vi "main.vi"() -> ()   [LabVIEW 2012]
uses:
  PCI9757_32.dll
panel:
  out "导入文件大小":dbl
  out "通道使能数组":dbl[](array[numeric])
  out "通道量程数组":dbl[](array[numeric])
  out "通道总数":dbl
  out "数组":path[](array[path])
  in  "退出系统":bool
  in  "选项卡控件":enum32{"AD采集", "数据回放"}(tab)
  in  "时钟源选择":u16(ring) items=["内部时钟", "外部时钟"]
  in  "触发方向":u16(ring) items=["负向触发", "正向触发", "正负向触发"]
  in  "触发类型":u16(ring) items=["边沿触发", "脉冲触发"]
  in  "触发源信号":u16(ring) items=["ATR触发", "DTR触发源"]
  in  "触发模式":u16(ring) items=["软件内触发", "硬件后触发"]
  out "混合信号图":dbl[][](graph)
  in  "通道3":bool
  in  "通道2":bool
  in  "通道1":bool
  in  "通道0":bool
  in  "停止AD":bool
  in  "开始AD":bool
  in  "存储":bool
  out "状态":u8(slide) scale=0.0..10.0
  in  "通道0量程":u16(ring) items=["-10000mV~+10000mV", "-5000mV~+5000mV", "-2500mV~+2500mV", "0-10000mV", "0-5000mV"]
  in  "通道3量程":u16(ring) items=["-10000mV~10000mV", "-5000mV~+5000mV", "-2500mV~+2500mV", "0-10000mV", "0-5000mV"]
  in  "通道1量程":u16(ring) items=["-10000mV~+10000mV", "-5000mV~+5000mV", "-2500mV~+2500mV", "0-10000mV", "0-5000mV"]
  in  "通道2量程":u16(ring) items=["-10000mV~+10000mV", "-5000mV~+5000mV", "-2500mV~+2500mV", "0-10000mV", "0-5000mV"]
  in  "文件名":string
  in  "触发电平":u32
  in  "触发灵敏窗":u32=40
  in  "测试功能":enum16{"非空", "半满", "DMA"}(ring)
  in  "采样频率":u32=10000
  in  "导入":bool
  out "Waveform Graph 3":dynamicdata(graph)
  in  "开始":bool
  in  "刷新速度":u32(knob)=100 min=100 max=1000 step=100 scale=100.0..1000.0
  in  "显示点数":u32(knob)=1000 min=1 max=10000 step=1000 scale=1.0..10000.0
  in  "量程输入":i32(ring) items=["±10000mV", "±5000mV", "±2500mV", "0-10000mV", "0-5000mV"]
  # "通道使能"
  # "通道量程"
  # "mV"
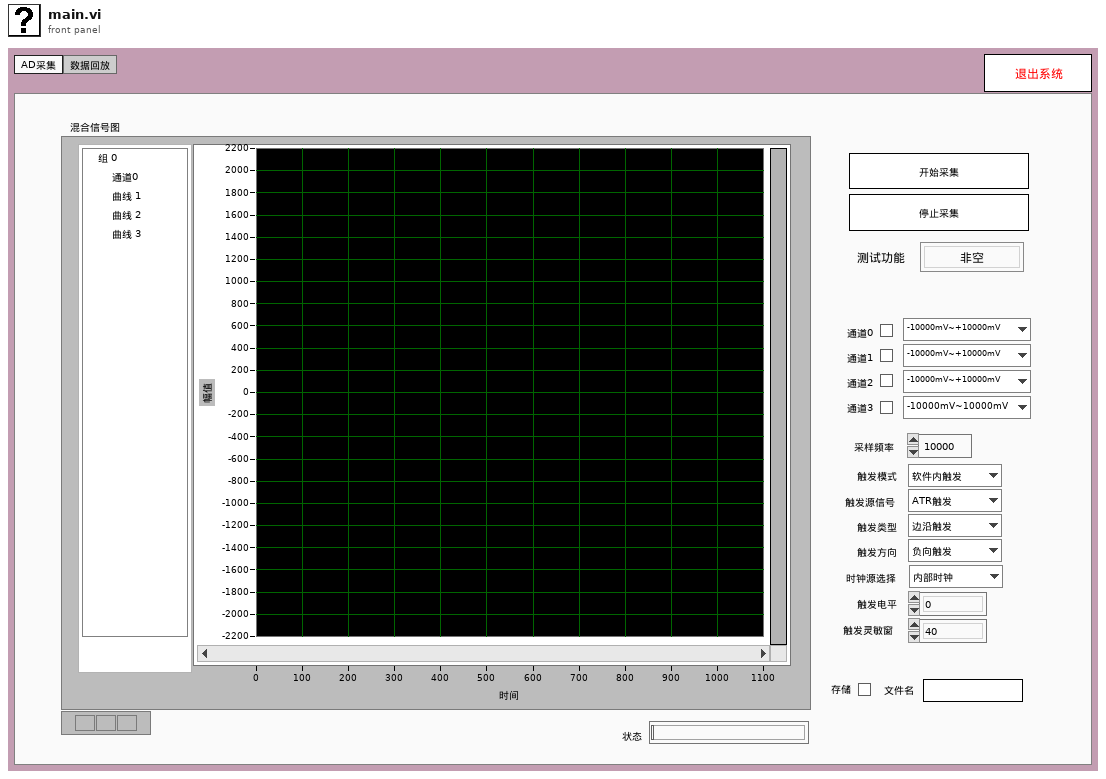
[diagram p1: front panel]
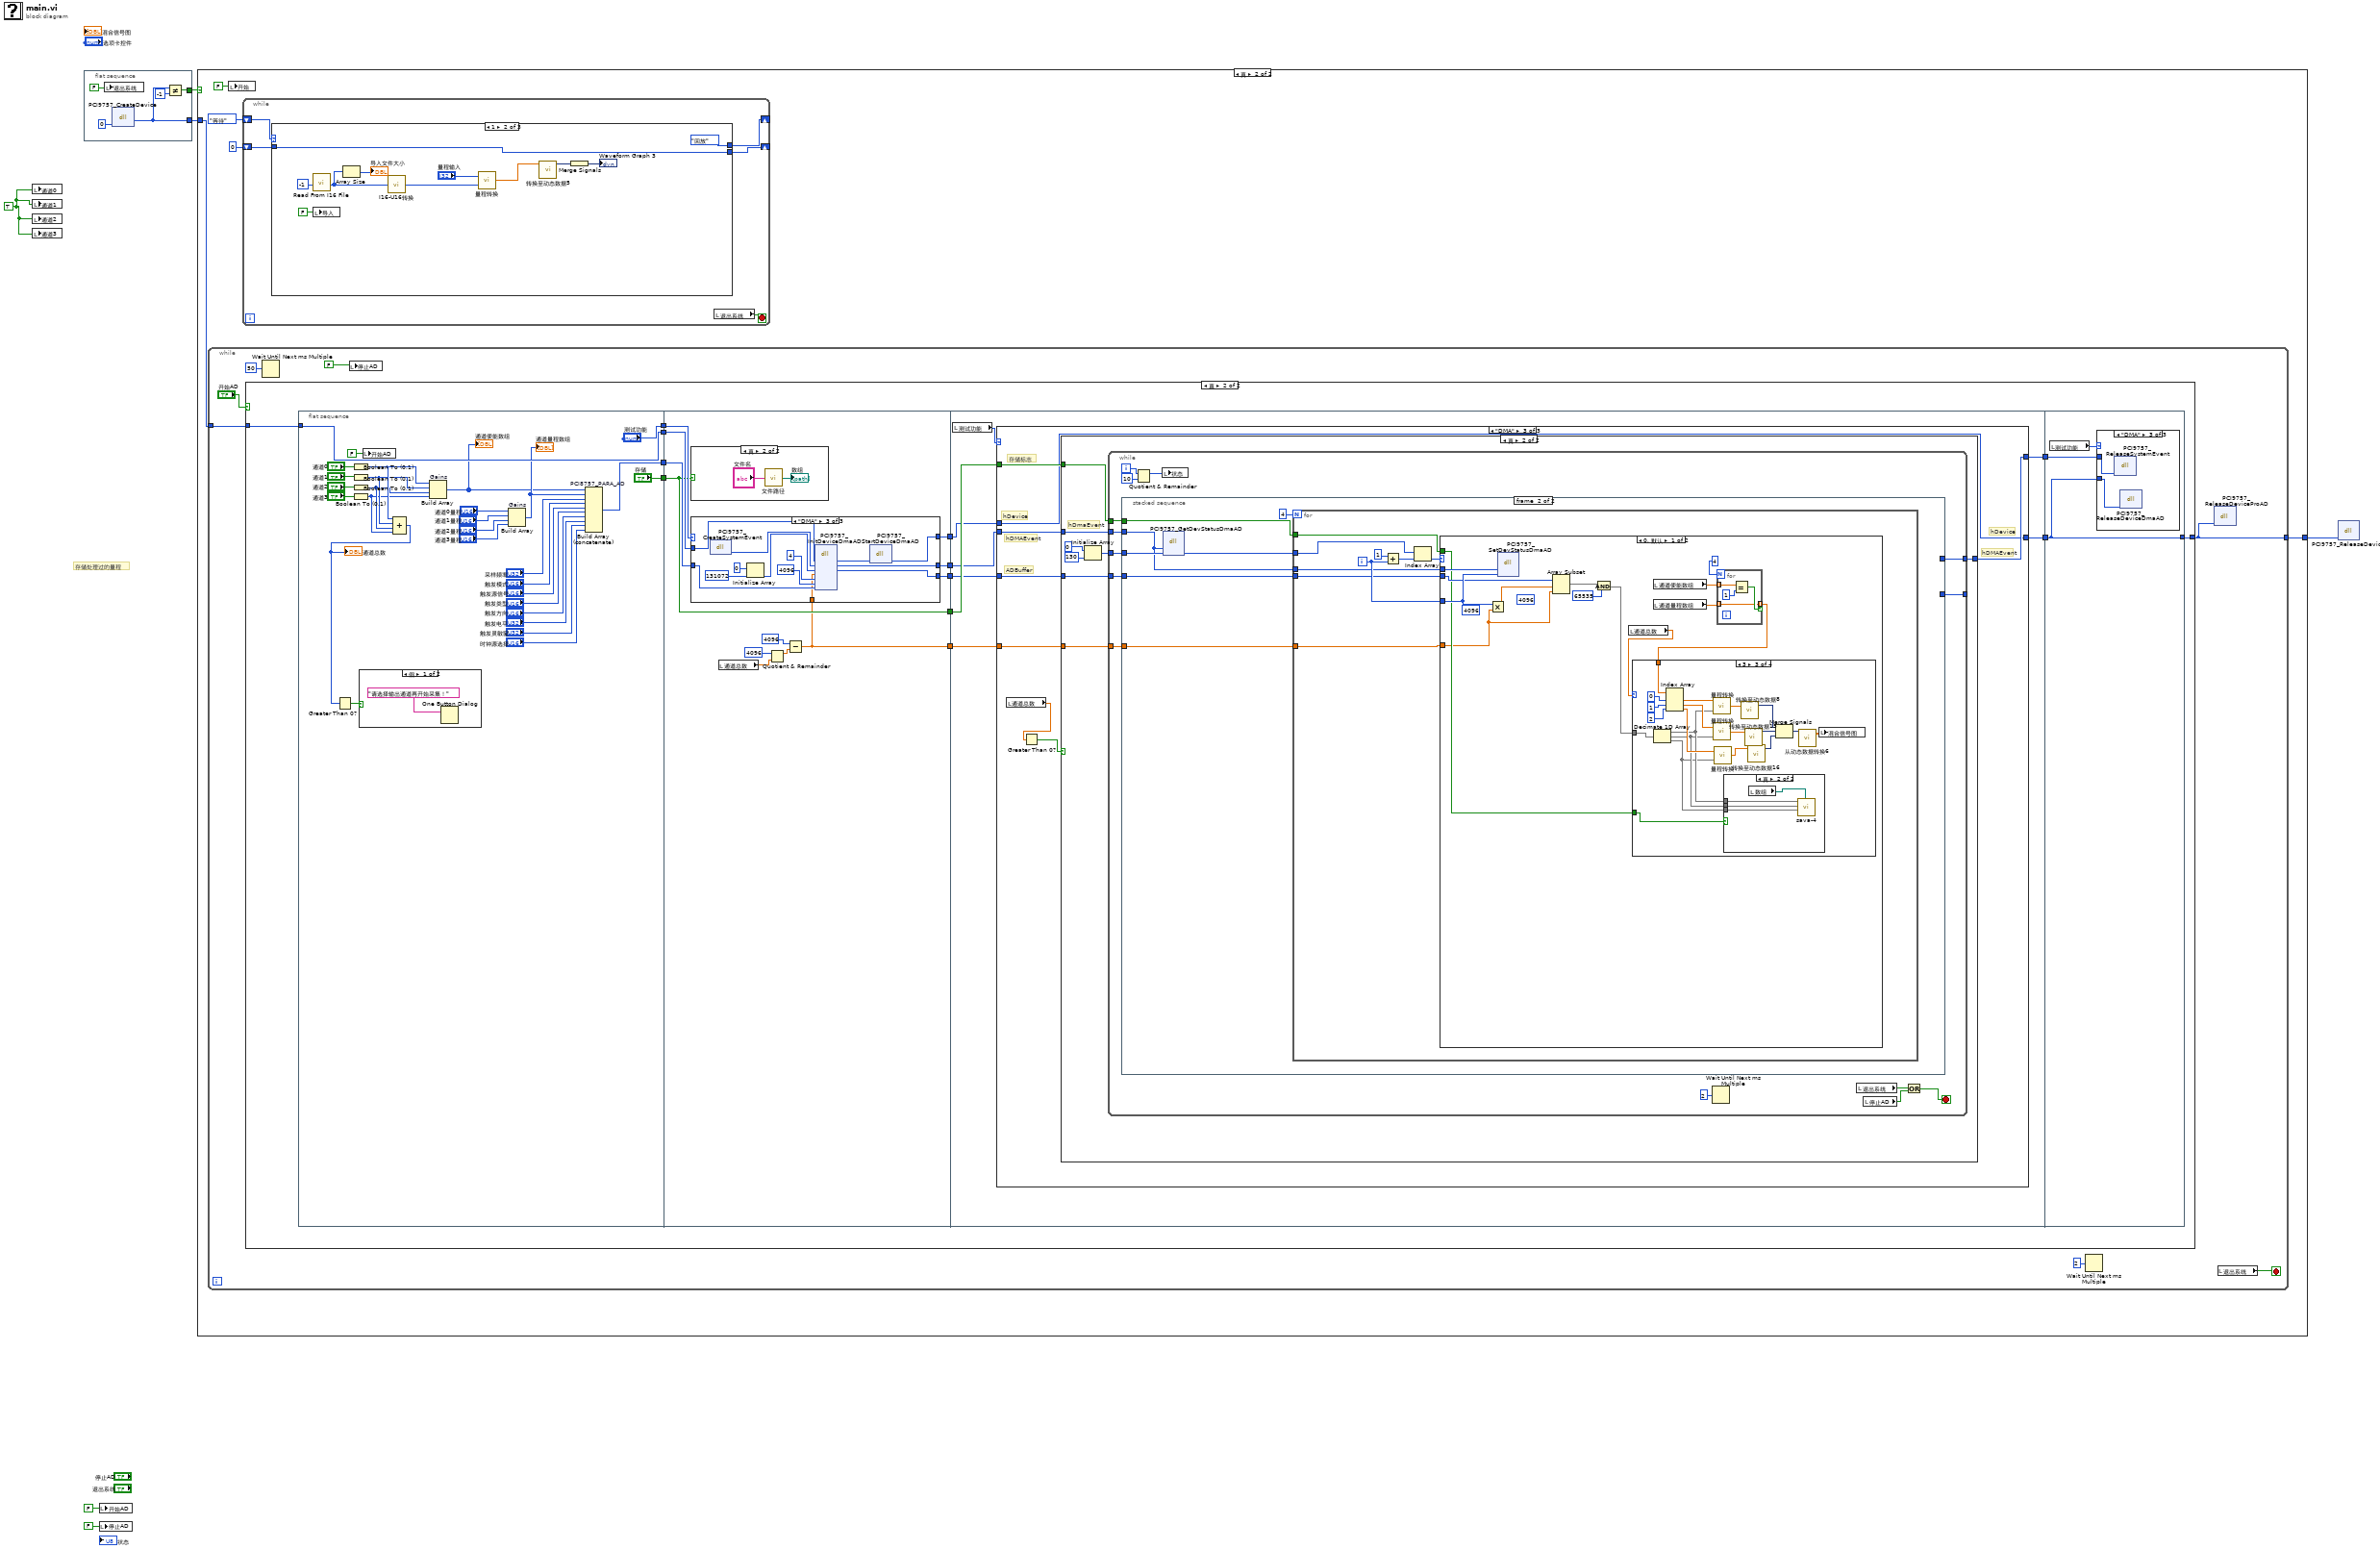
[diagram p0: block diagram]
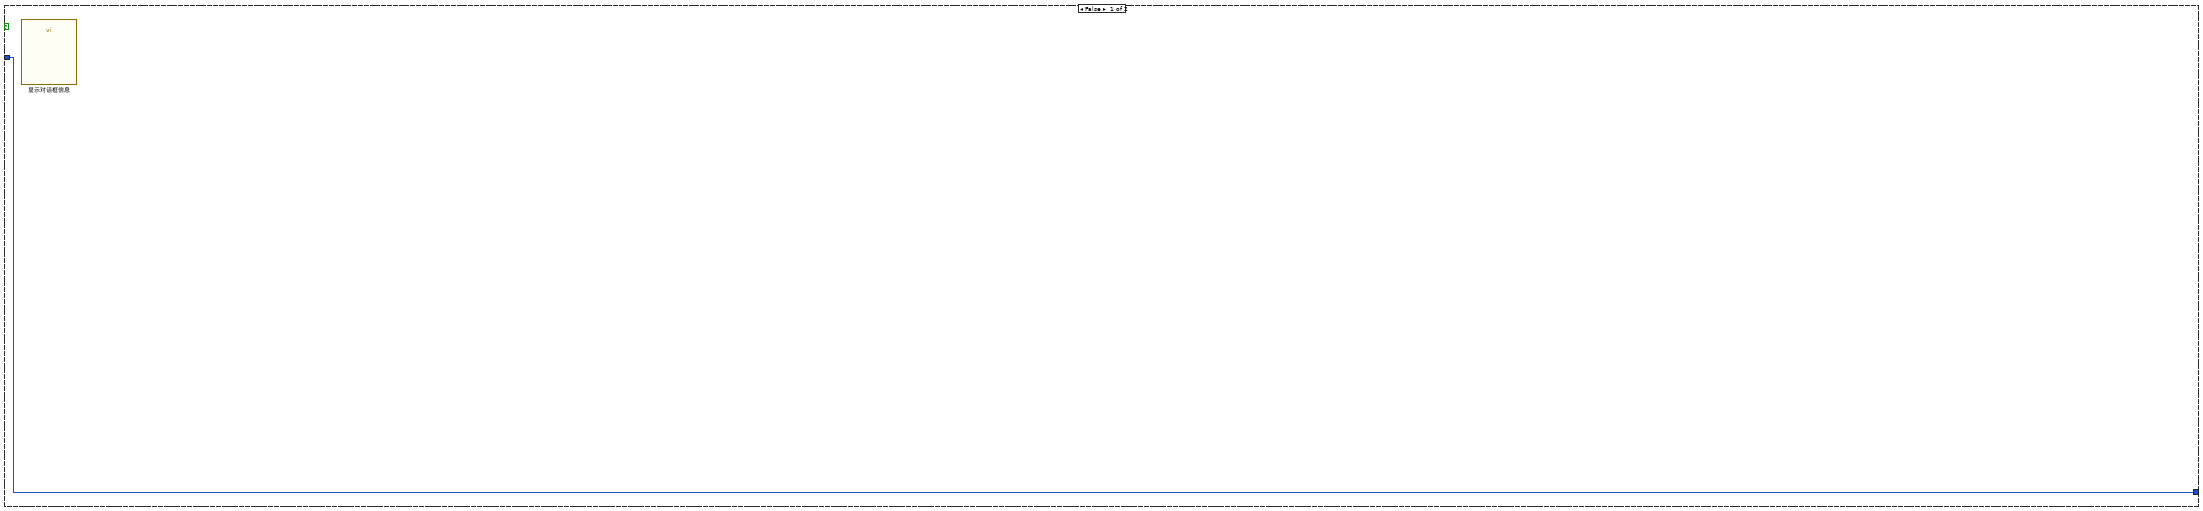
[diagram p2: hidden frame]
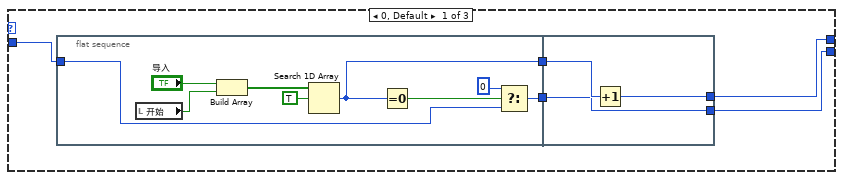
[diagram p3: hidden frame]
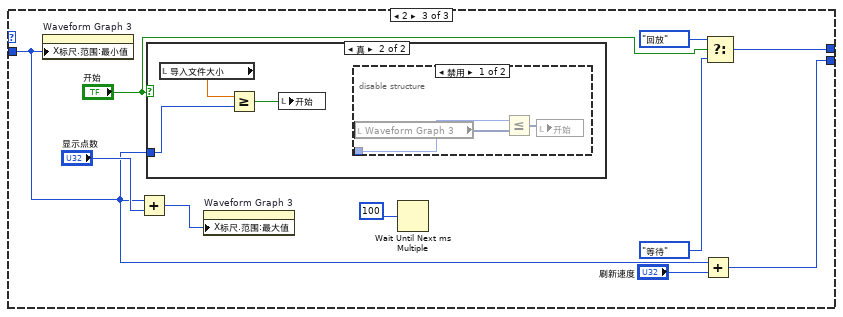
[diagram p4: hidden frame]
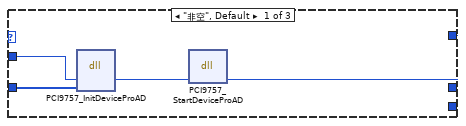
[diagram p10: hidden frame]
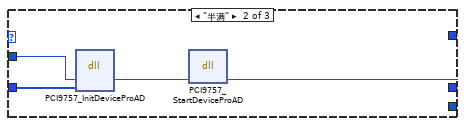
[diagram p11: hidden frame]
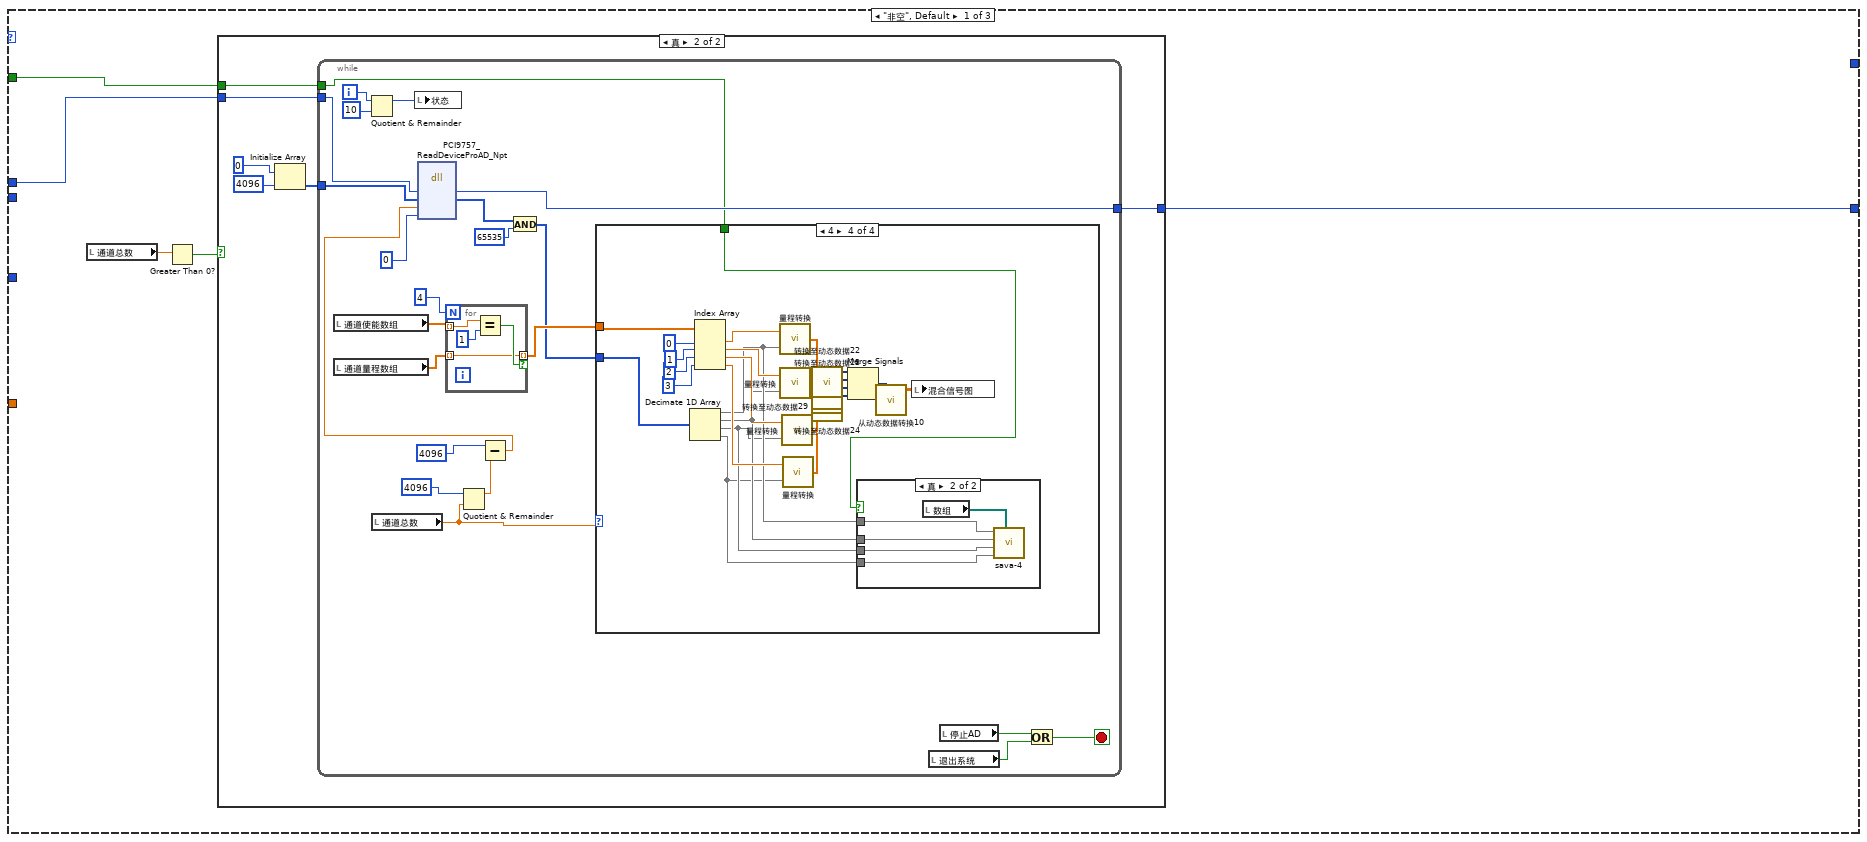
[diagram p12: hidden frame]
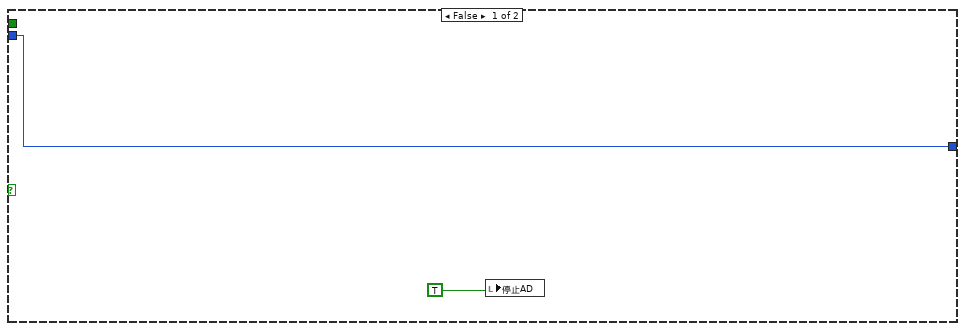
[diagram p13: hidden frame]
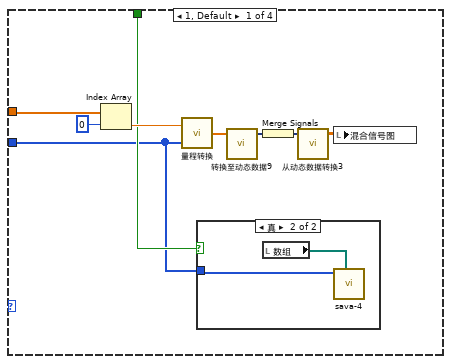
[diagram p14: hidden frame]
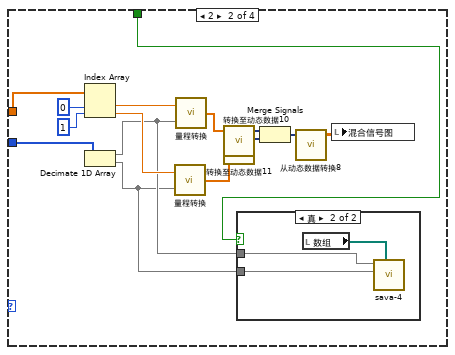
[diagram p16: hidden frame]
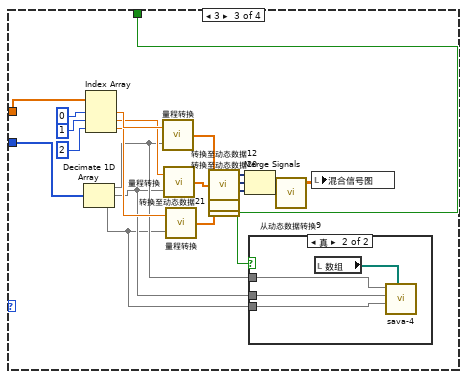
[diagram p18: hidden frame]
diagram:
  w1 = TRUE
  # "存储处理过的量程"
  n1 = local write "通道0"(w1) -> ()
  n2 = local write "通道1"(w1) -> ()
  n3 = local write "通道2"(w1) -> ()
  n4 = local write "通道3"(w1) -> ()
  n5 = flat-sequence {
    tunnel: [w10] -> w4
    tunnel: [w8] -> w3
    frame #0 {
      n6 = local write "退出系统"(FALSE ("退出系统")) -> ()
      n7 = dll-call lib="PCI9757_32.dll" fn="PCI9757_CreateDevice" label="CreateDevice"("DeviceID"=0) -> ("返回类型"=w8:i32)  [unwired: 4 in, 2 out]
      n8 = Not Equal?(x=w8, y=-1) -> (x != y?=w10:bool)
    }
  }
  n9 = local write "开始AD"(FALSE ("开始AD")) -> ()
  n10 = local write "停止AD"(FALSE ("停止AD")) -> ()
  n11 = case shown="真" w4 {
    tunnel: w3 -> [w12 w14]
    tunnel: [w12 w13] -> w2
    frame False {
      n12 = call "显示对话框信息"() -> ()  [unwired: 10 in, 2 out]
    }
    frame True {
      n13 = while {
        tunnel: w14 -> [w70]
        tunnel: [w69] -> w13
        stop <- w71 stop-if-true
        n14 = case shown="真" "开始AD" {
          tunnel: w70 -> [w74 w82]
          tunnel: [w74 w80] -> w69
          frame False {
          }
          frame True {
            n15 = flat-sequence {
              tunnel: ["测试功能"] -> w87
              tunnel: ["存储"] -> w85
              tunnel: [w109] -> w84
              tunnel: [w114] -> w83
              tunnel: w82 -> [w114]
              tunnel: [w124] -> w86
              tunnel: w87 -> [w129]
              tunnel: w85 -> [w123]
              tunnel: w84 -> [w128]
              tunnel: w83 -> [w127]
              tunnel: [w123] -> w79
              tunnel: [w126] -> w78
              tunnel: [w125] -> w77
              tunnel: [w118] -> w75
              tunnel: w86 -> [w158]
              tunnel: [w160] -> w81
              tunnel: w79 -> [w159]
              tunnel: w78 -> [w157]
              tunnel: w77 -> [w156]
              tunnel: [w154] -> w76
              tunnel: w75 -> [w153]
              tunnel: w81 -> [w588]
              tunnel: [w588] -> w80
              tunnel: w76 -> [w587]
              frame #0 {
                n16 = Boolean To (0,1)(Boolean="通道0") -> (0, 1=w96:i16)
                n17 = Boolean To (0,1)(Boolean="通道1") -> (0, 1=w95:i16)
                n18 = Boolean To (0,1)(Boolean="通道2") -> (0, 1=w94:i16)
                n19 = Boolean To (0,1)(Boolean="通道3") -> (0, 1=w93:i16)
                n20 = local write "开始AD"(FALSE ("开始AD")) -> ()
                n21 = Compound Arithmetic op=ADD(w96, w95, w94, w93) -> (w92:i16)
                "通道总数" <- w92
                n22 = Greater Than 0?(x=w92) -> (x > 0?=w97:bool)
                n23 = case shown="假" w97 {
                  frame False {
                    n24 = One Button Dialog(message="请选择输出通道再开始采集！") -> ()  [unwired: 1 in, 1 out]
                  }
                  frame True {
                  }
                }
                n25 = Build Array "Gains"(w96, w95, w94, w93) -> (w90:i16[])
                "通道使能数组" <- w90
                n26 = Build Array "Gains"("通道0量程", "通道1量程", "通道2量程", "通道3量程") -> (w91:u16[])
                "通道量程数组" <- w91
                n27 = Build Array (concatenate) "PCI8757_PARA_AD"(w90, w91, "采样频率", "触发模式", "触发源信号", "触发类型", "触发方向", "触发电平", "触发灵敏窗", "时钟源选择") -> (w109:u32[])
              }
              frame #1 {
                n28 = case shown="真" w123 {
                  frame False {
                  }
                  frame True {
                    n29 = call "文件路径.vi"("文件名"="文件名") -> ("数组"=→"数组":path[])
                  }
                }
                n30 = local read "通道总数"() -> (w120:dbl)
                n31 = Quotient & Remainder(x=4096 ("nReadSizeWords"), y=w120) -> (x-y*floor(x/y)=w119:dbl)  [unwired: 1 out]
                n32 = Subtract(x=4096 ("nReadSizeWords"), y=w119) -> (x-y=w118:dbl)
                n33 = case shown="\"DMA\"" w129 {
                  tunnel: w128 -> [w133 w137 w143]
                  tunnel: w127 -> [w134 w138 w141]
                  tunnel: [_ _ w145] -> w126
                  tunnel: [_ _ w144] -> w125
                  tunnel: [w132 w136 w142] -> w124
                  tunnel: w118 -> [_ _ w140]
                  frame "非空", Default {
                    n34 = dll-call lib="PCI9757_32.dll" fn="PCI9757_InitDeviceProAD" label="InitDeviceProAD"("hDevice"=w134, "pAPara"=w133) -> ("hDevice"=w135:i32)  [unwired: 5 in, 2 out]
                    n35 = dll-call lib="PCI9757_32.dll" fn="PCI9757_StartDeviceProAD" label="StartDeviceProAD"("hDevice"=w135) -> ("hDevice"=w132:i32)  [unwired: 4 in, 2 out]
                  }
                  frame "半满" {
                    n36 = dll-call lib="PCI9757_32.dll" fn="PCI9757_InitDeviceProAD" label="InitDeviceProAD"("hDevice"=w138, "pAPara"=w137) -> ("hDevice"=w139:i32)  [unwired: 5 in, 2 out]
                    n37 = dll-call lib="PCI9757_32.dll" fn="PCI9757_StartDeviceProAD" label="StartDeviceProAD"("hDevice"=w139) -> ("hDevice"=w136:i32)  [unwired: 4 in, 2 out]
                  }
                  frame "DMA" {
                    n38 = dll-call lib="PCI9757_32.dll" fn="PCI9757_CreateSystemEvent" label="CreateSystemEvent"() -> ("hEvent"=w149:i32)  [unwired: 3 in, 2 out]
                    n39 = Initialize Array(0, 131072 ("dimension size")) -> (w148:i32[])
                    n40 = dll-call lib="PCI9757_32.dll" fn="PCI9757_InitDeviceDmaAD" label="InitDeviceDmaAD"("hDevice"=w141, "hDmaEvent"=w149, "ADBuffer"=w148, "nReadSizeWords"=w140, "nSegmentCount"=4, "nSegmentSizeWords"=4096, "pADPara"=w143) -> ("hDevice"=w152:i32, "hDmaEvent"=w145:i32, "ADBuffer"=w144:u32[])  [unwired: 8 in, 2 out]
                    n41 = dll-call lib="PCI9757_32.dll" fn="PCI9757_StartDeviceDmaAD" label="StartDeviceDmaAD"("hDevice"=w152) -> ("hDevice"=w142:i32)  [unwired: 4 in, 2 out]
                  }
                }
              }
              frame #2 {
                n42 = local read "测试功能"() -> (w155:enum16{"非空", "半满", "DMA"})
                n43 = case shown="\"DMA\"" w155 {
                  tunnel: w158 -> [w165 w287 w430]
                  tunnel: [w164 w284 w430] -> w160
                  tunnel: w159 -> [w163 w288 w431]
                  tunnel: w157 -> [_ _ w433]
                  tunnel: w156 -> [_ _ w429]
                  tunnel: [_ _ w432] -> w154
                  tunnel: w153 -> [_ _ w426]
                  frame "非空", Default {
                    n44 = local read "通道总数"() -> (w162:dbl)
                    n45 = Greater Than 0?(x=w162) -> (x > 0?=w161:bool)
                    n46 = case shown="真" w161 {
                      tunnel: w165 -> [w167 w170]
                      tunnel: [w167 w169] -> w164
                      tunnel: w163 -> [_ w168]
                      frame False {
                        n47 = local write "停止AD"(TRUE) -> ()
                      }
                      frame True {
                        n48 = Initialize Array(0, 4096 ("dimension size")) -> (w171:i32[])
                        n49 = while {
                          tunnel: w171 -> [w188]
                          tunnel: w170 -> [w187]
                          tunnel: [w186] -> w169
                          tunnel: w168 -> [w179]
                          i -> [w192]
                          stop <- w194 stop-if-true
                          n50 = local read "通道使能数组"() -> (w183:dbl[])
                          n51 = local read "通道量程数组"() -> (w182:dbl[])
                          n52 = Quotient & Remainder(x=w192, y=10) -> (x-y*floor(x/y)=w191:i32)  [unwired: 1 out]
                          n53 = local read "通道总数"() -> (w177:dbl)
                          n54 = local write "状态"(w191) -> ()
                          n55 = for {
                            N: 4 -> [_]
                            tunnel: w183 -> [w283] mode=indexing
                            tunnel: w182 -> [w280] mode=indexing
                            tunnel: [w280] -> w181 mode=indexing if=w281
                            n56 = Equal?(x=w283, y=1) -> (x = y?=w281:bool)
                          }
                          n57 = Quotient & Remainder(x=4096, y=w177) -> (x-y*floor(x/y)=w176:dbl)  [unwired: 1 out]
                          n58 = Subtract(x=4096, y=w176) -> (x-y=w174:dbl)
                          n59 = dll-call lib="PCI9757_32.dll" fn="PCI9757_ReadDeviceProAD_Npt" label="ReadDeviceProAD_Npt"("hDevice"=w187, "ADBuffer"=w188, "nReadSizeWords"=w174, "nRetSizeWords"=0) -> ("hDevice"=w186:i32, "ADBuffer"=w185:u32[])  [unwired: 6 in, 2 out]
                          n60 = And(x=w185, y=65535) -> (x .and. y?=w180:u32[])
                          n61 = case shown="4" w177 {
                            tunnel: w181 -> [w205 w222 w245 w274]
                            tunnel: w180 -> [w197 w219 w241 w269]
                            tunnel: w179 -> [w198 w208 w226 w250]
                            frame 1, Default {
                              n62 = Index Array(array=w205, index=0) -> (element=w203:dbl)
                              n63 = call "量程转换.vi"("输入"=w197, "量程输入"=w203) -> ("输出"=w200:dbl[])
                              n64 = case shown="真" w198 {
                                tunnel: w197 -> [_ w206]
                                frame False {
                                }
                                frame True {
                                n65 = local read "数组"() -> (w207:path[])
                                n66 = call "sava-4.vi"("datafile"=w207, "1D array"=w206) -> ()  [unwired: 10 in]
                                }
                              }
                              n67 = call "转换至动态数据9"("Array"=w200) -> ("Dynamic Data Type"=w199:dynamicdata)  [unwired: 3 in]
                              n68 = Merge Signals(w199) -> (w202:dynamicdata)
                              n69 = call "从动态数据转换3"("Dynamic Data Type"=w202) -> ("Array"=w201:dbl[][])  [unwired: 3 in]
                              n70 = local write "混合信号图"(w201) -> ()
                            }
                            frame 2 {
                              n71 = Index Array(array=w222, index #1=0, index #2=1) -> (element #1=w218:dbl, element #2=w217:dbl)
                              n72 = Decimate 1D Array(w219) -> (w210:u32[], w209:u32[])
                              n73 = call "量程转换.vi"("输入"=w209, "量程输入"=w217) -> ("输出"=w214:dbl[])
                              n74 = call "量程转换.vi"("输入"=w210, "量程输入"=w218) -> ("输出"=w216:dbl[])
                              n75 = call "转换至动态数据10"("Array"=w216) -> ("Dynamic Data Type"=w215:dynamicdata)  [unwired: 3 in]
                              n76 = call "转换至动态数据11"("Array"=w214) -> ("Dynamic Data Type"=w213:dynamicdata)  [unwired: 3 in]
                              n77 = case shown="真" w208 {
                                tunnel: w210 -> [_ w224]
                                tunnel: w209 -> [_ w223]
                                frame False {
                                }
                                frame True {
                                n78 = local read "数组"() -> (w225:path[])
                                n79 = call "sava-4.vi"("datafile"=w225, "1D array 2"=w223, "1D array"=w224) -> ()  [unwired: 9 in]
                                }
                              }
                              n80 = Merge Signals(w215, w213) -> (w212:dynamicdata)
                              n81 = call "从动态数据转换8"("Dynamic Data Type"=w212) -> ("Array"=w211:dbl[][])  [unwired: 3 in]
                              n82 = local write "混合信号图"(w211) -> ()
                            }
                            frame 3 {
                              n83 = Decimate 1D Array(w241) -> (w229:u32[], w228:u32[], w227:u32[])
                              n84 = Index Array(array=w245, index #1=0, index #2=1, index #3=2) -> (element #1=w240:dbl, element #2=w239:dbl, element #3=w238:dbl)
                              n85 = call "量程转换.vi"("输入"=w229, "量程输入"=w240) -> ("输出"=w237:dbl[])
                              n86 = call "量程转换.vi"("输入"=w228, "量程输入"=w239) -> ("输出"=w235:dbl[])
                              n87 = call "量程转换.vi"("输入"=w227, "量程输入"=w238) -> ("输出"=w233:dbl[])
                              n88 = call "转换至动态数据12"("Array"=w237) -> ("Dynamic Data Type"=w236:dynamicdata)  [unwired: 3 in]
                              n89 = call "转换至动态数据20"("Array"=w235) -> ("Dynamic Data Type"=w234:dynamicdata)  [unwired: 3 in]
                              n90 = call "转换至动态数据21"("Array"=w233) -> ("Dynamic Data Type"=w232:dynamicdata)  [unwired: 3 in]
                              n91 = Merge Signals(w236, w234, w232) -> (w231:dynamicdata)
                              n92 = case shown="真" w226 {
                                tunnel: w229 -> [_ w248]
                                tunnel: w228 -> [_ w247]
                                tunnel: w227 -> [_ w246]
                                frame False {
                                }
                                frame True {
                                n93 = local read "数组"() -> (w249:path[])
                                n94 = call "sava-4.vi"("datafile"=w249, "1D array 3"=w246, "1D array 2"=w247, "1D array"=w248) -> ()  [unwired: 8 in]
                                }
                              }
                              n95 = call "从动态数据转换9"("Dynamic Data Type"=w231) -> ("Array"=w230:dbl[][])  [unwired: 3 in]
                              n96 = local write "混合信号图"(w230) -> ()
                            }
                            frame 4 {
                              n97 = Decimate 1D Array(w269) -> (w254:u32[], w253:u32[], w252:u32[], w251:u32[])
                              n98 = Index Array(array=w274, index #1=0, index #2=1, index #3=2, index #4=3) -> (element #1=w268:dbl, element #2=w267:dbl, element #3=w266:dbl, element #4=w265:dbl)
                              n99 = call "量程转换.vi"("输入"=w254, "量程输入"=w268) -> ("输出"=w264:dbl[])
                              n100 = call "量程转换.vi"("输入"=w253, "量程输入"=w267) -> ("输出"=w262:dbl[])
                              n101 = call "量程转换.vi"("输入"=w252, "量程输入"=w266) -> ("输出"=w260:dbl[])
                              n102 = call "量程转换.vi"("输入"=w251, "量程输入"=w265) -> ("输出"=w258:dbl[])
                              n103 = call "转换至动态数据22"("Array"=w264) -> ("Dynamic Data Type"=w263:dynamicdata)  [unwired: 3 in]
                              n104 = call "转换至动态数据23"("Array"=w262) -> ("Dynamic Data Type"=w261:dynamicdata)  [unwired: 3 in]
                              n105 = call "转换至动态数据24"("Array"=w260) -> ("Dynamic Data Type"=w259:dynamicdata)  [unwired: 3 in]
                              n106 = call "转换至动态数据29"("Array"=w258) -> ("Dynamic Data Type"=w257:dynamicdata)  [unwired: 3 in]
                              n107 = Merge Signals(w263, w261, w259, w257) -> (w256:dynamicdata)
                              n108 = case shown="真" w250 {
                                tunnel: w254 -> [_ w278]
                                tunnel: w253 -> [_ w277]
                                tunnel: w252 -> [_ w276]
                                tunnel: w251 -> [_ w275]
                                frame False {
                                }
                                frame True {
                                n109 = local read "数组"() -> (w279:path[])
                                n110 = call "sava-4.vi"("datafile"=w279, "1D array 4"=w275, "1D array 3"=w276, "1D array 2"=w277, "1D array"=w278) -> ()  [unwired: 7 in]
                                }
                              }
                              n111 = call "从动态数据转换10"("Dynamic Data Type"=w256) -> ("Array"=w255:dbl[][])  [unwired: 3 in]
                              n112 = local write "混合信号图"(w255) -> ()
                            }
                          }
                          n113 = local read "退出系统"() -> (w196:bool)
                          n114 = local read "停止AD"() -> (w195:bool)
                          n115 = Or(x=w195, y=w196) -> (x .or. y?=w194:bool)
                        }
                      }
                    }
                  }
                  frame "半满" {
                    n116 = local read "通道总数"() -> (w285:dbl)
                    n117 = Greater Than 0?(x=w285) -> (x > 0?=w286:bool)
                    n118 = case shown="真" w286 {
                      tunnel: w288 -> [_ w293]
                      tunnel: w287 -> [w290 w292]
                      tunnel: [w290 w291] -> w284
                      frame False {
                        n119 = local write "停止AD"(TRUE) -> ()
                      }
                      frame True {
                        n120 = Initialize Array(0, 4096 ("dimension size")) -> (w294:i32[])
                        n121 = while {
                          tunnel: w292 -> [w301]
                          tunnel: w294 -> [w300]
                          tunnel: w293 -> [w299]
                          tunnel: [w297] -> w291
                          i -> [w303]
                          stop <- w306 stop-if-true
                          n122 = stacked-sequence {
                            tunnel: [_ w336] -> w297
                            tunnel: w301 -> [w307 w335]
                            tunnel: w300 -> [_ w334]
                            tunnel: w299 -> [_ w323]
                            frame #0 {
                              n123 = Initialize Array(0, 3) -> (w308:i32[])
                              n124 = while {
                                tunnel: w308 -> [w317]
                                tunnel: w307 -> [w311]
                                stop <- w312 stop-if-true
                                n125 = dll-call lib="PCI9757_32.dll" fn="PCI9757_GetDevStatusProAD" label="GetDevStatusProAD"("hDevice"=w311, "ADStatus"=w317) -> ("ADStatus"=w315:i32[])  [unwired: 5 in, 2 out]
                                n126 = Index Array(array=w315, index=2) -> (element=w314:i32)
                                n127 = Equal?(x=w314, y=1) -> (x = y?=w312:bool)
                              }
                            }
                            frame #1 {
                              n128 = local read "通道总数"() -> (w319:dbl)
                              n129 = Quotient & Remainder(x=4096, y=w319) -> (x-y*floor(x/y)=w321:dbl)  [unwired: 1 out]
                              n130 = Subtract(x=4096, y=w321) -> (x-y=w318:dbl)
                              n131 = Wait Until Next ms Multiple(millisecond multiple=u32 10) -> ()  [unwired: 1 out]
                              n132 = dll-call lib="PCI9757_32.dll" fn="PCI9757_ReadDeviceProAD_Half" label="ReadDeviceProAD_Half"("hDevice"=w335, "ADBuffer"=w334, "nReadSizeWords"=w318, "nRetSizeWords"=0) -> ("hDevice"=w336:i32, "ADBuffer"=w331:u32[])  [unwired: 6 in, 2 out]
                              n133 = local read "通道使能数组"() -> (w328:dbl[])
                              n134 = local read "通道量程数组"() -> (w327:dbl[])
                              n135 = Array Subset(array=w331, index=0, length=w318) -> (w330:u32[])
                              n136 = for {
                                N: 4 -> [_]
                                tunnel: w328 -> [w425] mode=indexing
                                tunnel: w327 -> [w422] mode=indexing
                                tunnel: [w422] -> w325 mode=indexing if=w423
                                n137 = Equal?(x=w425, y=1) -> (x = y?=w423:bool)
                              }
                              n138 = And(x=w330, y=65535) -> (x .and. y?=w324:u32[])
                              n139 = local read "通道总数"() -> (w326:dbl)
                              n140 = case shown="4" w326 {
                                tunnel: w325 -> [w347 w364 w387 w416]
                                tunnel: w324 -> [w340 w359 w383 w411]
                                tunnel: w323 -> [w339 w350 w368 w396]
                                frame 1, Default {
                                n141 = Index Array(array=w347, index=0) -> (element=w345:dbl)
                                n142 = call "量程转换.vi"("输入"=w340, "量程输入"=w345) -> ("输出"=w344:dbl[])
                                n143 = case shown="真" w339 {
                                tunnel: w340 -> [_ w348]
                                frame False {
                                }
                                frame True {
                                n144 = local read "数组"() -> (w349:path[])
                                n145 = call "sava-4.vi"("datafile"=w349, "1D array"=w348) -> ()  [unwired: 10 in]
                                }
                                }
                                n146 = call "转换至动态数据"("Array"=w344) -> ("Dynamic Data Type"=w343:dynamicdata)  [unwired: 3 in]
                                n147 = Merge Signals(w343) -> (w342:dynamicdata)
                                n148 = call "从动态数据转换"("Dynamic Data Type"=w342) -> ("Array"=w341:dbl[][])  [unwired: 3 in]
                                n149 = local write "混合信号图"(w341) -> ()
                                }
                                frame 2 {
                                n150 = Decimate 1D Array(w359) -> (w352:u32[], w351:u32[])
                                n151 = Index Array(array=w364, index #1=0, index #2=1) -> (element #1=w361:dbl, element #2=w360:dbl)
                                n152 = call "量程转换.vi"("输入"=w352, "量程输入"=w361) -> ("输出"=w358:dbl[])
                                n153 = call "量程转换.vi"("输入"=w351, "量程输入"=w360) -> ("输出"=w356:dbl[])
                                n154 = call "转换至动态数据2"("Array"=w358) -> ("Dynamic Data Type"=w357:dynamicdata)  [unwired: 3 in]
                                n155 = call "转换至动态数据3"("Array"=w356) -> ("Dynamic Data Type"=w355:dynamicdata)  [unwired: 3 in]
                                n156 = case shown="真" w350 {
                                tunnel: w352 -> [_ w366]
                                tunnel: w351 -> [_ w365]
                                frame False {
                                }
                                frame True {
                                n157 = local read "数组"() -> (w367:path[])
                                n158 = call "sava-4.vi"("datafile"=w367, "1D array 2"=w365, "1D array"=w366) -> ()  [unwired: 9 in]
                                }
                                }
                                n159 = Merge Signals(w357, w355) -> (w354:dynamicdata)
                                n160 = call "从动态数据转换11"("Dynamic Data Type"=w354) -> ("Array"=w353:dbl[][])  [unwired: 3 in]
                                n161 = local write "混合信号图"(w353) -> ()
                                }
                                frame 3 {
                                n162 = Decimate 1D Array(w383) -> (w371:u32[], w370:u32[], w369:u32[])
                                n163 = Index Array(array=w387, index #1=0, index #2=1, index #3=2) -> (element #1=w382:dbl, element #2=w381:dbl, element #3=w380:dbl)
                                n164 = call "量程转换.vi"("输入"=w371, "量程输入"=w382) -> ("输出"=w379:dbl[])
                                n165 = call "量程转换.vi"("输入"=w370, "量程输入"=w381) -> ("输出"=w377:dbl[])
                                n166 = call "量程转换.vi"("输入"=w369, "量程输入"=w380) -> ("输出"=w375:dbl[])
                                n167 = case shown="真" w368 {
                                tunnel: w371 -> [_ w390]
                                tunnel: w370 -> [_ w389]
                                tunnel: w369 -> [_ w388]
                                frame False {
                                }
                                frame True {
                                n168 = local read "数组"() -> (w391:path[])
                                n169 = call "sava-4.vi"("datafile"=w391, "1D array 3"=w388, "1D array 2"=w389, "1D array"=w390) -> ()  [unwired: 8 in]
                                }
                                }
                                n170 = call "转换至动态数据4"("Array"=w379) -> ("Dynamic Data Type"=w378:dynamicdata)  [unwired: 3 in]
                                n171 = call "转换至动态数据30"("Array"=w377) -> ("Dynamic Data Type"=w376:dynamicdata)  [unwired: 3 in]
                                n172 = call "转换至动态数据31"("Array"=w375) -> ("Dynamic Data Type"=w374:dynamicdata)  [unwired: 3 in]
                                n173 = Merge Signals(w378, w376, w374) -> (w373:dynamicdata)
                                n174 = call "从动态数据转换12"("Dynamic Data Type"=w373) -> ("Array"=w372:dbl[][])  [unwired: 3 in]
                                n175 = local write "混合信号图"(w372) -> ()
                                }
                                frame 4 {
                                n176 = Decimate 1D Array(w411) -> (w395:u32[], w394:u32[], w393:u32[], w392:u32[])
                                n177 = Index Array(array=w416, index #1=0, index #2=1, index #3=2, index #4=3) -> (element #1=w410:dbl, element #2=w409:dbl, element #3=w408:dbl, element #4=w407:dbl)
                                n178 = call "量程转换.vi"("输入"=w395, "量程输入"=w410) -> ("输出"=w406:dbl[])
                                n179 = call "量程转换.vi"("输入"=w394, "量程输入"=w409) -> ("输出"=w404:dbl[])
                                n180 = call "量程转换.vi"("输入"=w393, "量程输入"=w408) -> ("输出"=w402:dbl[])
                                n181 = call "量程转换.vi"("输入"=w392, "量程输入"=w407) -> ("输出"=w400:dbl[])
                                n182 = call "转换至动态数据32"("Array"=w406) -> ("Dynamic Data Type"=w405:dynamicdata)  [unwired: 3 in]
                                n183 = call "转换至动态数据33"("Array"=w404) -> ("Dynamic Data Type"=w403:dynamicdata)  [unwired: 3 in]
                                n184 = call "转换至动态数据34"("Array"=w402) -> ("Dynamic Data Type"=w401:dynamicdata)  [unwired: 3 in]
                                n185 = call "转换至动态数据35"("Array"=w400) -> ("Dynamic Data Type"=w399:dynamicdata)  [unwired: 3 in]
                                n186 = case shown="真" w396 {
                                tunnel: w395 -> [_ w420]
                                tunnel: w394 -> [_ w419]
                                tunnel: w393 -> [_ w418]
                                tunnel: w392 -> [_ w417]
                                frame False {
                                }
                                frame True {
                                n187 = local read "数组"() -> (w421:path[])
                                n188 = call "sava-4.vi"("datafile"=w421, "1D array 4"=w417, "1D array 3"=w418, "1D array 2"=w419, "1D array"=w420) -> ()  [unwired: 7 in]
                                }
                                }
                                n189 = Merge Signals(w405, w403, w401, w399) -> (w398:dynamicdata)
                                n190 = call "从动态数据转换13"("Dynamic Data Type"=w398) -> ("Array"=w397:dbl[][])  [unwired: 3 in]
                                n191 = local write "混合信号图"(w397) -> ()
                                }
                              }
                            }
                          }
                          n192 = Quotient & Remainder(x=w303, y=10) -> (x-y*floor(x/y)=w302:i32)  [unwired: 1 out]
                          n193 = local read "退出系统"() -> (w305:bool)
                          n194 = local read "停止AD"() -> (w298:bool)
                          n195 = local write "状态"(w302) -> ()
                          n196 = Or(x=w305, y=w298) -> (x .or. y?=w306:bool)
                        }
                      }
                    }
                  }
                  frame "DMA" {
                    # "hDMAEvent"
                    # "hDMAEvent"
                    # "hDevice"
                    # "ADBuffer"
                    # "存储标志"
                    # "hDevice"
                    n197 = local read "通道总数"() -> (w428:dbl)
                    n198 = Greater Than 0?(x=w428) -> (x > 0?=w427:bool)
                    n199 = case shown="真" w427 {
                      tunnel: w433 -> [w434 w441]
                      tunnel: w429 -> [_ w440]
                      tunnel: [w434 w438] -> w432
                      tunnel: w431 -> [_ w437]
                      tunnel: w426 -> [_ w436]
                      frame False {
                        n200 = local write "停止AD"(TRUE) -> ()
                      }
                      frame True {
                        # "hDmaEvent"
                        n201 = Initialize Array(0 ("element"), 130 ("dimension size")) -> (w439:i32[])
                        n202 = while {
                          tunnel: w439 -> [w457]
                          tunnel: w440 -> [w456]
                          tunnel: w441 -> [w455]
                          tunnel: [w454] -> _
                          tunnel: [w453] -> w438
                          tunnel: w437 -> [w449]
                          tunnel: w436 -> [w444]
                          i -> [w452]
                          stop <- w445 stop-if-true
                          n203 = stacked-sequence {
                            tunnel: w457 -> [_ w473]
                            tunnel: w456 -> [_ w475]
                            tunnel: w455 -> [w458 w472]
                            tunnel: [w458 _] -> w454
                            tunnel: [w459 _] -> w453
                            tunnel: w449 -> [_ w471]
                            tunnel: w444 -> [_ w470]
                            frame #0 {
                              n204 = while {
                                tunnel: [w464] -> w459
                                tunnel: w458 -> [w463]
                                stop <- w465 stop-if-true
                                n205 = dll-call lib="kernel32" fn="WaitForSingleObject"("hEvent"=w463, "dwMilliseconds"=100) -> ("返回类型"=w467:u32, "hEvent"=w464:i32)  [unwired: 4 in, 2 out]
                                n206 = Wait Until Next ms Multiple(millisecond multiple=u32 2 ("毫秒倍数")) -> ()  [unwired: 1 out]
                                n207 = local read "退出系统"() -> (w460:bool)
                                n208 = local read "停止AD"() -> (w462:bool)
                                n209 = Equal To 0?(x=w467) -> (x = 0?=w466:bool)
                                n210 = Compound Arithmetic op=OR(w466, w462, w460) -> (w465:bool)
                                n211 = Wait Until Next ms Multiple(millisecond multiple=u32 1) -> ()  [unwired: 1 out]
                              }
                            }
                            frame #1 {
                              n212 = dll-call lib="PCI9757_32" fn="PCI9757_GetDevStatusDmaAD" label="GetDevStatusDmaAD"("hDevice"=w472, "pDMAStatus"=w473) -> ("pDMAStatus"=w474:i32[])  [unwired: 5 in, 2 out]
                              n213 = for {
                                N: 4 -> [_]
                                tunnel: w474 -> [w480]
                                tunnel: w472 -> [w479]
                                tunnel: w475 -> [w481]
                                tunnel: w471 -> [w478]
                                tunnel: w470 -> [w477]
                                i -> [w483]
                                n214 = Add(x=1, y=w483) -> (x+y=w482:i32)
                                n215 = Index Array(array=w480, index=w482) -> (element=w485:i32)
                                n216 = case shown="0, 默认" w485 {
                                tunnel: w483 -> [w497 _]
                                tunnel: w479 -> [w498 _]
                                tunnel: w481 -> [w496 _]
                                tunnel: w478 -> [w487 _]
                                tunnel: w477 -> [w486 _]
                                frame 0, Default {
                                (unwired) 4096 ("y")
                                (unwired) 4096 ("length")
                                n217 = Multiply(x=w497, y=w486) -> (x*y=w499:dbl)
                                n218 = dll-call lib="PCI9757_32" fn="PCI9757_SetDevStatusDmaAD" label="SetDevStatusDmaAD"("hDevice"=w498, "iClrBufferID"=w497) -> ()  [unwired: 6 in, 2 out]
                                n219 = Array Subset(array=w496, index=w499, length=w486) -> (w494:u32[])
                                n220 = And(x=w494, y=65535) -> (x .and. y?=w488:u32[])
                                n221 = local read "通道总数"() -> (w489:dbl)
                                n222 = local read "通道使能数组"() -> (w492:dbl[])
                                n223 = local read "通道量程数组"() -> (w493:dbl[])
                                n224 = for {
                                N: 4 -> [_]
                                tunnel: w492 -> [w586] mode=indexing
                                tunnel: w493 -> [w583] mode=indexing
                                tunnel: [w583] -> w490 mode=indexing if=w584
                                n225 = Equal?(x=w586, y=1) -> (x = y?=w584:bool)
                                }
                                n226 = case shown="3" w489 {
                                tunnel: w490 -> [w508 w524 w544 w569]
                                tunnel: w488 -> [w500 w514 w543 w564]
                                tunnel: w487 -> [w501 w513 w529 w553]
                                frame 1, Default {
                                n227 = Index Array(array=w508, index=0) -> (element=w506:dbl)
                                n228 = call "量程转换.vi"("输入"=w500, "量程输入"=w506) -> ("输出"=w502:dbl[])
                                n229 = case shown="真" w501 {
                                tunnel: w500 -> [_ w509]
                                frame False {
                                }
                                frame True {
                                n230 = local read "数组"() -> (w510:path[])
                                n231 = call "sava-4.vi"("datafile"=w510, "1D array"=w509) -> ()  [unwired: 10 in]
                                }
                                }
                                n232 = call "转换至动态数据7"("Array"=w502) -> ("Dynamic Data Type"=w503:dynamicdata)  [unwired: 3 in]
                                n233 = Merge Signals(w503) -> (w505:dynamicdata)
                                n234 = call "从动态数据转换4"("Dynamic Data Type"=w505) -> ("Array"=w504:dbl[][])  [unwired: 3 in]
                                n235 = local write "混合信号图"(w504) -> ()
                                }
                                frame 2 {
                                n236 = Decimate 1D Array(w514) -> (w512:u32[], w511:u32[])
                                n237 = Index Array(array=w524, index #1=0, index #2=1) -> (element #1=w520:dbl, element #2=w519:dbl)
                                n238 = call "量程转换.vi"("输入"=w512, "量程输入"=w520) -> ("输出"=w525:dbl[])
                                n239 = call "量程转换.vi"("输入"=w511, "量程输入"=w519) -> ("输出"=w521:dbl[])
                                n240 = case shown="真" w513 {
                                tunnel: w512 -> [_ w527]
                                tunnel: w511 -> [_ w526]
                                frame False {
                                }
                                frame True {
                                n241 = local read "数组"() -> (w528:path[])
                                n242 = call "sava-4.vi"("datafile"=w528, "1D array 2"=w526, "1D array"=w527) -> ()  [unwired: 9 in]
                                }
                                }
                                n243 = call "转换至动态数据6"("Array"=w525) -> ("Dynamic Data Type"=w518:dynamicdata)  [unwired: 3 in]
                                n244 = call "转换至动态数据14"("Array"=w521) -> ("Dynamic Data Type"=w517:dynamicdata)  [unwired: 3 in]
                                n245 = Merge Signals(w518, w517) -> (w516:dynamicdata)
                                n246 = call "从动态数据转换5"("Dynamic Data Type"=w516) -> ("Array"=w515:dbl[][])  [unwired: 3 in]
                                n247 = local write "混合信号图"(w515) -> ()
                                }
                                frame 3 {
                                n248 = Decimate 1D Array(w543) -> (w532:u32[], w531:u32[], w530:u32[])
                                n249 = Index Array(array=w544, index #1=0, index #2=1, index #3=2) -> (element #1=w541:dbl, element #2=w540:dbl, element #3=w539:dbl)
                                n250 = call "量程转换.vi"("输入"=w532, "量程输入"=w541) -> ("输出"=w547:dbl[])
                                n251 = call "量程转换.vi"("输入"=w531, "量程输入"=w540) -> ("输出"=w538:dbl[])
                                n252 = call "量程转换.vi"("输入"=w530, "量程输入"=w539) -> ("输出"=w536:dbl[])
                                n253 = case shown="真" w529 {
                                tunnel: w532 -> [_ w551]
                                tunnel: w531 -> [_ w550]
                                tunnel: w530 -> [_ w549]
                                frame False {
                                }
                                frame True {
                                n254 = local read "数组"() -> (w552:path[])
                                n255 = call "sava-4.vi"("datafile"=w552, "1D array 3"=w549, "1D array 2"=w550, "1D array"=w551) -> ()  [unwired: 8 in]
                                }
                                }
                                n256 = call "转换至动态数据8"("Array"=w547) -> ("Dynamic Data Type"=w548:dynamicdata)  [unwired: 3 in]
                                n257 = call "转换至动态数据15"("Array"=w538) -> ("Dynamic Data Type"=w537:dynamicdata)  [unwired: 3 in]
                                n258 = call "转换至动态数据16"("Array"=w536) -> ("Dynamic Data Type"=w535:dynamicdata)  [unwired: 3 in]
                                n259 = Merge Signals(w548, w537, w535) -> (w534:dynamicdata)
                                n260 = call "从动态数据转换6"("Dynamic Data Type"=w534) -> ("Array"=w533:dbl[][])  [unwired: 3 in]
                                n261 = local write "混合信号图"(w533) -> ()
                                }
                                frame 4 {
                                n262 = Decimate 1D Array(w564) -> (w557:u32[], w556:u32[], w555:u32[], w554:u32[])
                                n263 = Index Array(array=w569, index #1=0, index #2=1, index #3=2, index #4=3) -> (element #1=w568:dbl, element #2=w567:dbl, element #3=w566:dbl, element #4=w565:dbl)
                                n264 = call "量程转换.vi"("输入"=w557, "量程输入"=w568) -> ("输出"=w575:dbl[])
                                n265 = call "量程转换.vi"("输入"=w556, "量程输入"=w567) -> ("输出"=w563:dbl[])
                                n266 = call "量程转换.vi"("输入"=w555, "量程输入"=w566) -> ("输出"=w561:dbl[])
                                n267 = call "量程转换.vi"("输入"=w554, "量程输入"=w565) -> ("输出"=w559:dbl[])
                                n268 = call "转换至动态数据13"("Array"=w575) -> ("Dynamic Data Type"=w576:dynamicdata)  [unwired: 3 in]
                                n269 = call "转换至动态数据17"("Array"=w563) -> ("Dynamic Data Type"=w562:dynamicdata)  [unwired: 3 in]
                                n270 = call "转换至动态数据18"("Array"=w561) -> ("Dynamic Data Type"=w560:dynamicdata)  [unwired: 3 in]
                                n271 = call "转换至动态数据19"("Array"=w559) -> ("Dynamic Data Type"=w558:dynamicdata)  [unwired: 3 in]
                                n272 = case shown="真" w553 {
                                tunnel: w557 -> [_ w581]
                                tunnel: w556 -> [_ w580]
                                tunnel: w555 -> [_ w579]
                                tunnel: w554 -> [_ w578]
                                frame False {
                                }
                                frame True {
                                n273 = local read "数组"() -> (w582:path[])
                                n274 = call "sava-4.vi"("datafile"=w582, "1D array 4"=w578, "1D array 3"=w579, "1D array 2"=w580, "1D array"=w581) -> ()  [unwired: 7 in]
                                }
                                }
                                n275 = Merge Signals(w576, w562, w560, w558) -> (w577:dynamicdata)
                                n276 = call "从动态数据转换7"("Dynamic Data Type"=w577) -> ("Array"=w574:dbl[][])  [unwired: 3 in]
                                n277 = local write "混合信号图"(w574) -> ()
                                }
                                }
                                }
                                frame 1 {
                                }
                                }
                              }
                            }
                          }
                          n278 = Quotient & Remainder(x=w452, y=10) -> (x-y*floor(x/y)=w450:i32)  [unwired: 1 out]
                          n279 = local write "状态"(w450) -> ()
                          n280 = Wait Until Next ms Multiple(millisecond multiple=u32 2 ("毫秒倍数")) -> ()  [unwired: 1 out]
                          n281 = local read "退出系统"() -> (w447:bool)
                          n282 = local read "停止AD"() -> (w446:bool)
                          n283 = Or(x=w447, y=w446) -> (x .or. y?=w445:bool)
                        }
                      }
                    }
                  }
                }
              }
              frame #3 {
                n284 = local read "测试功能"() -> (w589:enum16{"非空", "半满", "DMA"})
                n285 = case shown="\"DMA\"" w589 {
                  tunnel: w588 -> [w590 w591 w593]
                  tunnel: w587 -> [_ _ w592]
                  frame "非空", Default {
                    n286 = dll-call lib="PCI9757_32.dll" fn="PCI9757_ReleaseDeviceProAD" label="ReleaseDeviceProAD"("hDevice"=w590) -> ()  [unwired: 5 in, 2 out]
                  }
                  frame "半满" {
                    n287 = dll-call lib="PCI9757_32.dll" fn="PCI9757_ReleaseDeviceProAD" label="ReleaseDeviceProAD"("hDevice"=w591) -> ()  [unwired: 5 in, 2 out]
                  }
                  frame "DMA" {
                    n288 = dll-call lib="PCI9757_32.dll" fn="PCI9757_ReleaseSystemEvent" label="ReleaseSystemEvent"("hDmaEvent"=w592) -> ()  [unwired: 5 in, 2 out]
                    n289 = dll-call lib="PCI9757_32.dll" fn="PCI9757_ReleaseDeviceDmaAD" label="StopDeviceDmaAD"("hDevice"=w593) -> ()  [unwired: 5 in, 2 out]
                  }
                }
              }
            }
          }
        }
        n290 = Wait Until Next ms Multiple(millisecond multiple=u32 50 ("毫秒倍数")) -> ()  [unwired: 1 out]
        n291 = local write "停止AD"(FALSE) -> ()
        n292 = Wait Until Next ms Multiple(millisecond multiple=u32 2 ("毫秒倍数")) -> ()  [unwired: 1 out]
        n293 = dll-call lib="PCI9757_32.dll" fn="PCI9757_ReleaseDeviceProAD" label="ReleaseDeviceProAD"("hDevice"=w69) -> ()  [unwired: 5 in, 2 out]
        n294 = local read "退出系统"() -> (w71:bool)
      }
      n295 = local write "开始"(FALSE ("开始")) -> ()
      n296 = while {
        shift-right: [w20] -> _
        shift-left: 0 -> [w18]
        shift-right: [w21] -> _
        shift-left: enum16{"等待", "导入", "回放", "停止"}."等待" -> [w22]
        stop <- w19 stop-if-true
        n297 = case shown="1" w22 {
          tunnel: [w26 enum16{"等待", "导入", "回放", "停止"}."回放" w58] -> w21
          tunnel: w18 -> [w25 w49 w55]
          tunnel: [w23 w49 w56] -> w20
          frame 0, Default {
            n298 = flat-sequence {
              tunnel: [w31] -> w27
              tunnel: w25 -> [w30]
              tunnel: [w29] -> w24
              tunnel: w27 -> [w39]
              tunnel: [w38] -> w26
              tunnel: [w37] -> w23
              tunnel: w24 -> [w37]
              frame #0 {
                n299 = local read "开始"() -> (w33:bool)
                n300 = Build Array("导入", w33) -> (w35:bool[])
                n301 = Search 1D Array(1D array=w35, element=TRUE) -> (index of element=w31:i32)  [unwired: 1 in]
                n302 = Equal To 0?(x=w31) -> (x = 0?=w28:bool)
                n303 = Select(t=0, s=w28, f=w30) -> (s? t:f=w29:u32)
              }
              frame #1 {
                n304 = Increment(x=w39) -> (x+1=w38:i32)
              }
            }
          }
          frame 1 {
            n305 = call <vilib>:"Read From I16 File.vi"("2D number of columns/1D count (all as 1D:-1)"=-1) -> ("1D array"=w46:i16[])  [unwired: 6 in, 4 out]
            n306 = local write "导入"(FALSE ("导入")) -> ()
            n307 = Array Size(array=w46) -> (size(s)=→"导入文件大小":i32)
            n308 = call "I16-U16转换.vi"("输入"=w46) -> ("输出"=w42:i32[])
            n309 = call "量程转换.vi"("输入"=w42, "量程输入"="量程输入") -> ("输出"=w45:dbl[])
            n310 = call "转换至动态数据5"("Array"=w45) -> ("Dynamic Data Type"=w44:dynamicdata)  [unwired: 3 in]
            n311 = Merge Signals(w44) -> (→"Waveform Graph 3":dynamicdata)
          }
          frame 2 {
            n312 = property on="Waveform Graph 3" class="WFGraph (严格)"("X标尺.范围:最小值"=w55) -> ()  [unwired: 2 in, 2 out]
            n313 = Add(x=w55, y="显示点数") -> (x+y=w57:u32)
            n314 = case shown="真" "开始" {
              tunnel: w55 -> [_ w62]
              frame False {
              }
              frame True {
                n315 = local read "导入文件大小"() -> (w63:dbl)
                n316 = Greater Or Equal?(x=w63, y=w62) -> (x >= y?=w61:bool)
                n317 = local write "开始"(w61) -> ()
                n318 = disable-structure shown="禁用" {
                  disable-tunnel: _ -> [w66 _]
                  frame Disabled {
                    n319 = local read "Waveform Graph 3"() -> (w64:dynamicdata)
                    n320 = Less Or Equal?(x=w66, y=w64) -> (x <= y?=w65:dynamicdata)
                    n321 = local write "开始"(w65) -> ()
                  }
                  frame Enabled {
                  }
                }
              }
            }
            n322 = property on="Waveform Graph 3" class="WFGraph (严格)"("X标尺.范围:最大值"=w57) -> ()  [unwired: 2 in, 2 out]
            n323 = Wait Until Next ms Multiple(millisecond multiple=100) -> ()  [unwired: 1 out]
            n324 = Add(x=w55, y="刷新速度") -> (x+y=w56:u32)
            n325 = Select(t=enum16{"等待", "导入", "回放", "停止"}."回放", s="开始", f=enum16{"等待", "导入", "回放", "停止"}."等待") -> (s? t:f=w58:enum16{"等待", "导入", "回放", "停止"})
          }
        }
        n326 = local read "退出系统"() -> (w19:bool)
      }
    }
  }
  n327 = dll-call lib="PCI9757_32.dll" fn="PCI9757_ReleaseDevice" label="ReleaseDevice"("hDevice"=w2) -> ()  [unwired: 5 in, 2 out]
